vi "Index.vi"(8 "error in (no error)":errorcluster, 10 "Index":i32, 11 "Boolean Array in":refnum<class "Boolean Array.lvclass">) -> (0 "error out":errorcluster, 3 "Indexed element":refnum<class "Generic Data.lvclass">)   [LabVIEW 2020, in "Data.lvlib" / "Boolean Array.lvclass"]
doc: "Index an element from 'Generic Data in'.\nThis implementation returns a generic Boolean class with the indexed boolean."
uses:
  Boolean Array.lvclass
  Generic Data.lvclass
  Boolean Array.lvclass/Boolean Array.ctl
  Boolean/Boolean.lvclass/Boolean.ctl
  Boolean/Boolean.lvclass
  C:/Users/Henri/OneDrive/LabVIEW/Framework/Data/Generic Data/Generic Data.lvclass
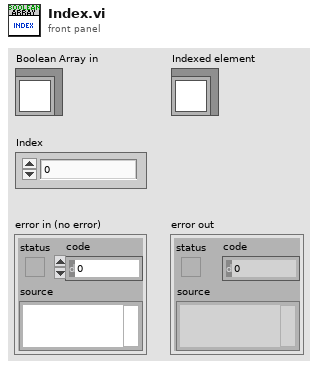
[diagram p1: front panel]
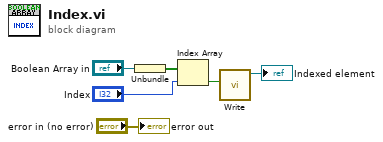
[diagram p0: block diagram]
diagram:
  n1 = Unbundle("Boolean Array in") -> (w5:bool[])
  n2 = Index Array(array=w5, index="Index") -> (element=w2:bool)
  n3 = call "Write.vi"("Boolean"=w2) -> ("Boolean out"=→"Indexed element":refnum<class "Boolean.lvclass">)  [unwired: 10 in]
  "error out" <- "error in (no error)"
